vi "Zoom Increment.vi"(11 "Range":T1) -> (3 "Increment":dbl)   [LabVIEW 2021, in "RocketPlot.lvlib"]
uses:
  RocketPlot.lvlib
  <vilib>/Utility/miscctls.llb/LVRangeTypeDef.ctl
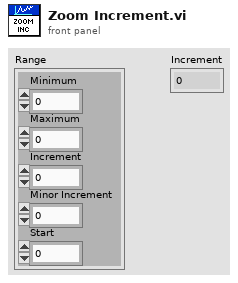
[diagram p1: front panel]
types:
  T1 = typedef "LVRangeTypeDef.ctl" = cluster{"Minimum":dbl, "Maximum":dbl, "Increment":dbl, "Minor Increment":dbl, "Start":dbl}
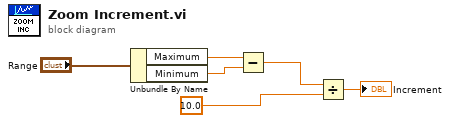
[diagram p0: block diagram]
diagram:
  n1 = Unbundle By Name("Range") -> ("Maximum"=w5:dbl, "Minimum"=w4:dbl)
  n2 = Subtract(x=w5, y=w4) -> (x-y=w3:dbl)
  n3 = Divide(x=w3, y=10.0) -> (x/y=→"Increment":dbl)
